vi "hpcnc move to position.vi"(0 "VISA Refnum in":refnum<visa-resource-name>, 1 "X":dbl, 2 "Y":dbl, 3 "Z":dbl, 4 "Speed":i32=100, 5 "error in":errorcluster) -> (14 "VISA Refnum out":refnum<visa-resource-name>, 19 "error out":errorcluster)   [LabVIEW 2014]
uses:
  HPCNC.lvlib
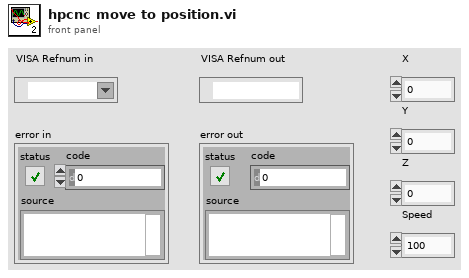
[diagram p1: front panel]
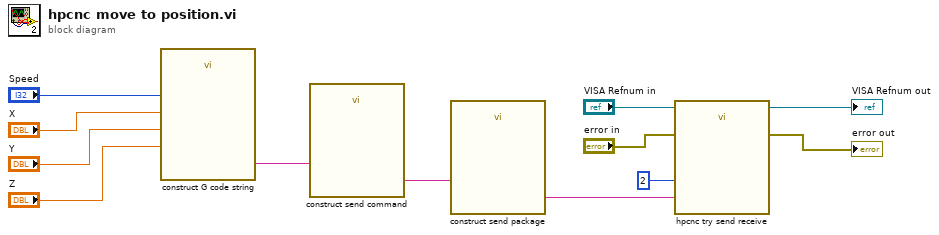
[diagram p0: block diagram]
diagram:
  n1 = call "construct G code string.vi"("Speed"="Speed", "ZF"="Z", "YF"="Y", "XF"="X") -> ("GCode"=w3:string)  [unwired: 5 in]
  n2 = call "construct send command.vi"("GCode"=w3) -> ("SendCommand"=w1:string)  [unwired: 9 in]
  n3 = call "construct send package.vi"("Send command"=w1) -> ("Send package"=w4:string)  [unwired: 8 in, 2 out]
  n4 = call "hpcnc try send receive.vi"("error in (no error)"="error in", "Max try number"=2, "Send package"=w4, "VISA Refnum in"="VISA Refnum in") -> ("error out"=→"error out":errorcluster, "VISA Refnum out"=→"VISA Refnum out":refnum<visa-resource-name>)  [unwired: 4 in, 2 out]
